vi "Volt Reader Trigger7.vi"() -> ()   [LabVIEW 2014]
uses:
  <vilib>/Utility/error.llb/DialogType.ctl
  <vilib>/_DAQmxBase/Internals/DAQmxBase Create Channel (AI-Voltage-Basic).vi
  <vilib>/_DAQmxBase/Internals/DAQmxBase Timing (Sample Clock).vi
  <vilib>/measure/mamon.llb/Trigger Detection for 1 Channel.vi
  <vilib>/_DAQmxBase/Internals/DAQmxBase Read (Analog 2D DBL NChan NSamp).vi
  <vilib>/measure/NI_MAPro.lvlib
panel:
  in  "Polarity":bool
  out "size of output array":i32
  out "Buffer Full?":bool
  out "trigger location":dbl format="%#_2g"
  out "Waveform Graph 2":waveform(dbl)(graph)
  in  "Continue Graphing":bool
  in  "Knob amplifier":dbl
  in  "Enable Center":bool
  in  "Center Button":bool
  in  "Knob":dbl(knob) scale=0.0..1.0
  out "Waveform Graph":waveform(dbl)(graph)
  in  "Buffer (Seconds)":dbl
  out "Threshold":dbl
  in  "units":i32(ring)=10348 items=["Volts"=10348, "From Custom Scale"=10065]
  in  "stop":bool
  in  "physical channels":tag
  in  "maximum value":dbl=5.0 format="%0.2f"
  in  "minimum value":dbl=-5.0 format="%0.2f"
  in  "rate":i32=1000 caption="Sample Rate"
  # "The inputs above MUST BE\nPreset before running"
  # "NOTE: Just change the Y axis value"
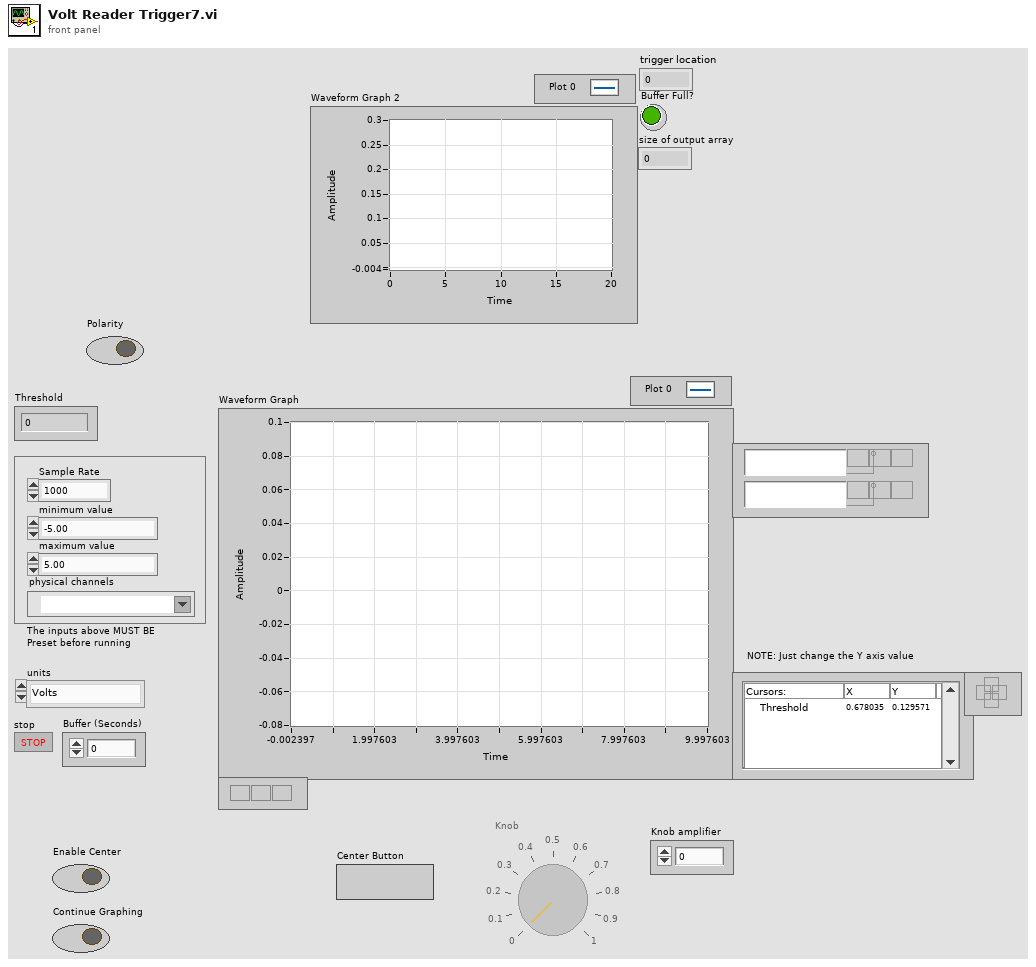
[diagram p1: front panel]
types:
  T1 = enum8{"Enabled", "Disabled", "Disabled and Grayed Out"}
  T2 = typedef "DialogType.ctl" = u16
  T3 = typedef "LVCursorListTypeDef.ctl" = cluster{"Name":string, "Color":u32, "Style":u8, "Point Style":u8, "Name Visible":bool, "Allow Drag":bool, "Cursor Mode":u32, "Plot":i32, "Index":i32, "Position":cluster{"X":dbl, "Y":dbl}, "X Scale":u32, "Y Scale":u32, "Watch Plots":i32[], "Watch All Plots":bool, "Plot Area":i32, "Label Offset":cluster{"X":dbl, "Y":dbl}}[]
  T4 = cluster{"Name":string, "Color":u32, "Style":u8, "Point Style":u8, "Name Visible":bool, "Allow Drag":bool, "Cursor Mode":u32, "Plot":i32, "Index":i32, "Position":cluster{"X":dbl, "Y":dbl}, "X Scale":u32, "Y Scale":u32, "Watch Plots":i32[], "Watch All Plots":bool, "Plot Area":i32, "Label Offset":cluster{"X":dbl, "Y":dbl}}
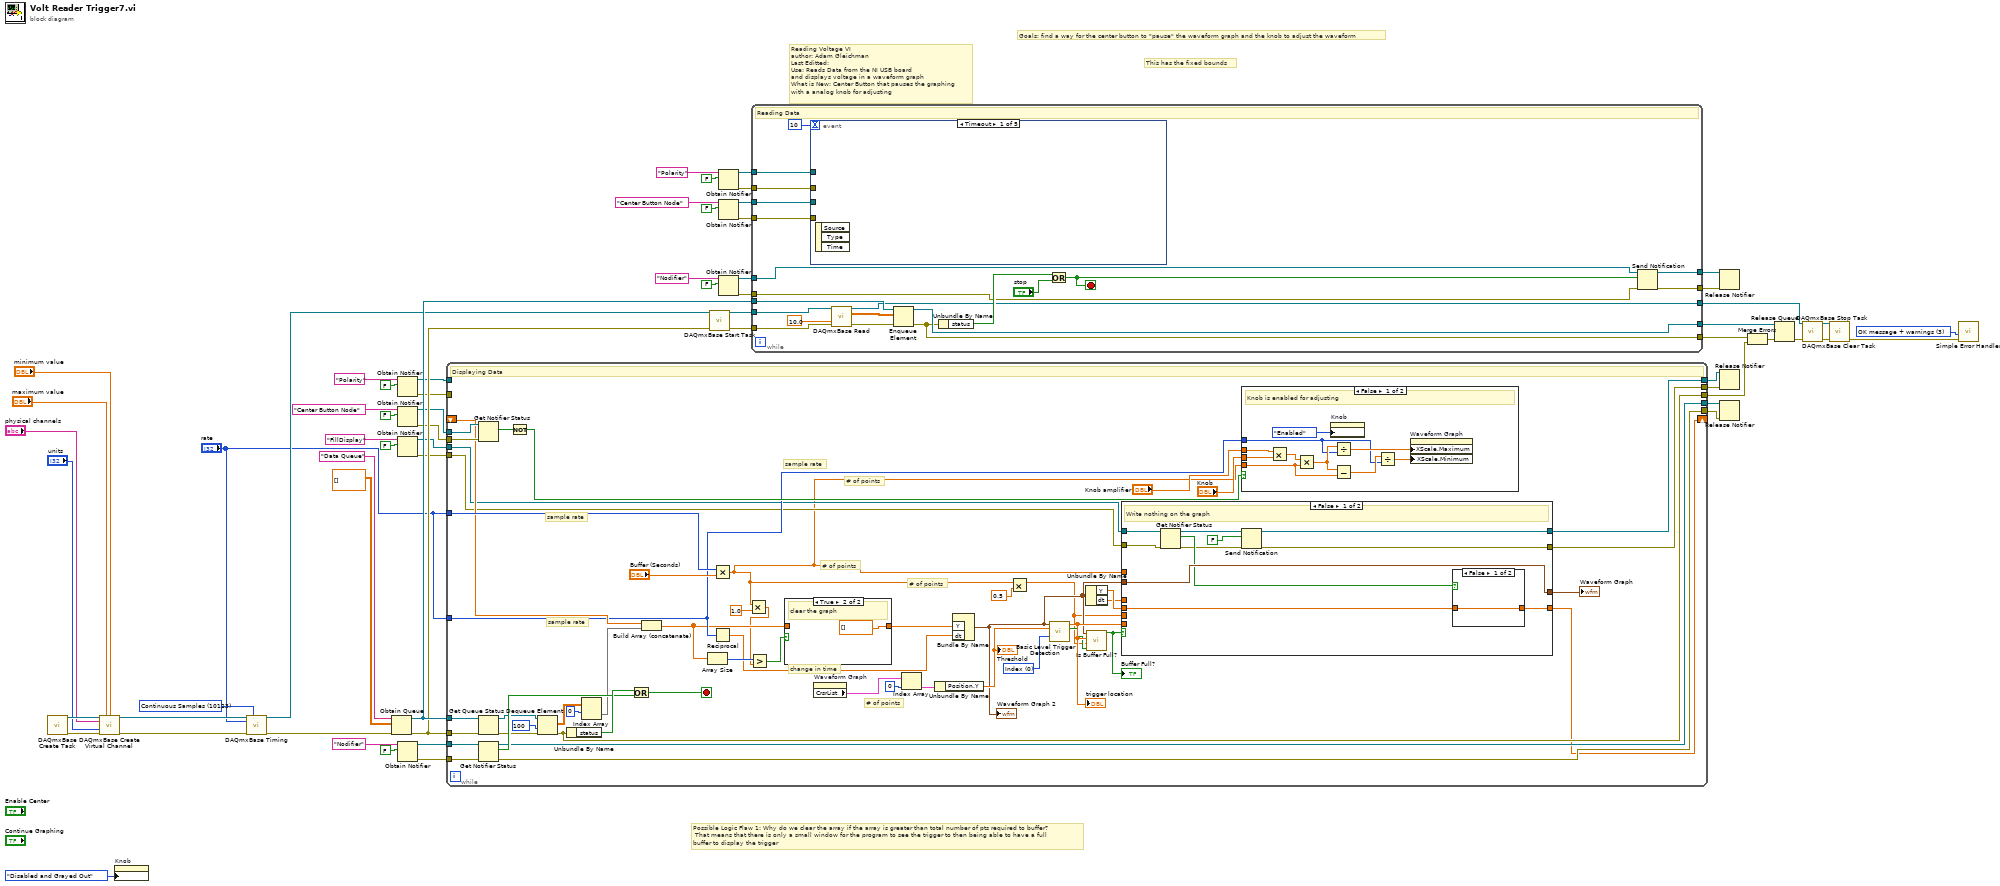
[diagram p0: block diagram]
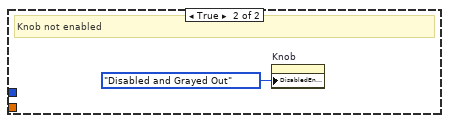
[diagram p3: hidden frame]
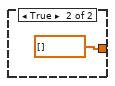
[diagram p4: hidden frame]
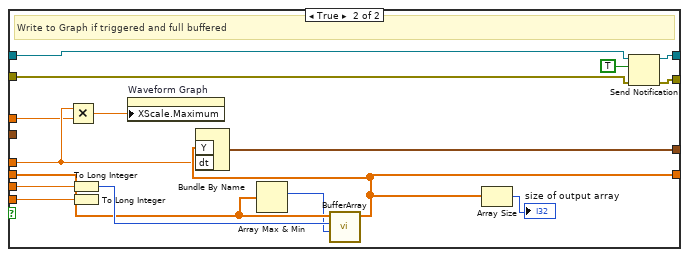
[diagram p5: hidden frame]
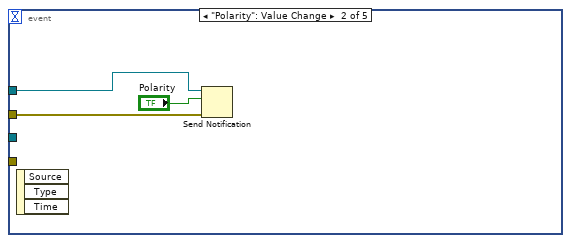
[diagram p6: hidden frame]
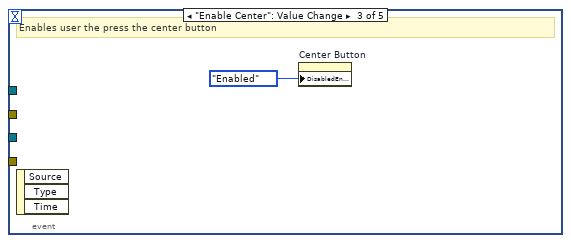
[diagram p7: hidden frame]
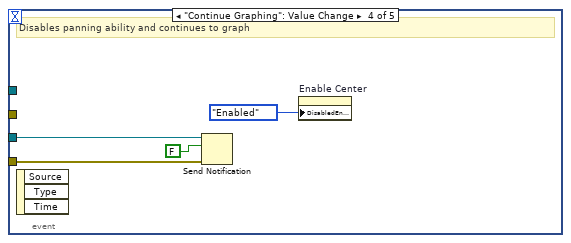
[diagram p8: hidden frame]
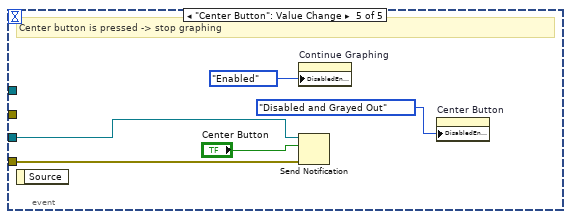
[diagram p9: hidden frame]
diagram:
  w40 = 10123 items=["Finite Samples"=10178, "Continuous Samples"=10123, "Hardware Timed Single Point"=12522] ("sample mode")
  w42 = T2 3 items=["no dialog", "OK message", "continue or stop message", "OK message + warnings", "continue/stop + warnings"] ("type of dialog (OK msg:1)")
  # "Possible Logic Flaw 1: Why do we clear the array if the array is greater than total number of pts required to buffer?\n That means that there is only a small window for the program to see the trigger to then being able to have a full\nbuffer to display the trigger"
  # "Goals: find a way for the center button to \"pause\" the waveform graph and the knob to adjust the waveform"
  # "This has the fixed bounds"
  # "Reading Voltage VI\nauthor: Adam Gleichman\nLast Editted: \nUse: Reads Data from the NI USB board\nand displays voltage in a waveform graph\nWhat is New: Center Button that pauses the graphing\nwith a analog knob for adjusting"
  n1 = call <vilib>:"DAQmxBase Create Task.vi"() -> ("task out"=w62:refnum<k21>, "error out"=w61:errorcluster)  [unwired: 5 in, 9 out]
  n2 = call-poly <vilib>:"DAQmxBase Create Virtual Channel.vi"("task in"=w62, "maximum value"="maximum value", "minimum value"="minimum value", "physical channels"="physical channels", "units"="units", "error in"=w61) -> ("task out"=w59:refnum<k21>, "error out"=w60:errorcluster)  [unwired: 3 in, 5 out]
  n3 = property on="Knob" class="Knob (strict)"("DisabledEnum"=T1."Disabled and Grayed Out" ("Disabled")) -> ()  [unwired: 2 in, 2 out]
  n4 = call-poly <vilib>:"DAQmxBase Timing.vi"("task/channels in"=w59, "sample mode"=w40, "rate"="rate", "error in"=w60) -> ("task out"=w28:refnum<k21>, "error out"=w27:errorcluster)  [unwired: 3 in, 7 out]
  n5 = Obtain Queue(name (unnamed)="Data Queue", element data type=dbl[][] [] ("data"), error in (no error)=w27) -> (queue out=w49:refnum<queue>, error out=w48:errorcluster)  [unwired: 2 in, 1 out]
  n6 = Obtain Notifier(name (unnamed)="Polarity", notification data type=FALSE) -> (notifier out=w8:refnum<notifier>, error out=w7:errorcluster)  [unwired: 2 in, 1 out]
  n7 = Obtain Notifier(name (unnamed)="Center Button Node", notification data type=FALSE) -> (notifier out=w15:refnum<notifier>, error out=w19:errorcluster)  [unwired: 2 in, 1 out]
  n8 = Obtain Notifier(name (unnamed)="FillDisplay", notification data type=FALSE) -> (notifier out=w6:refnum<notifier>, error out=w5:errorcluster)  [unwired: 2 in, 1 out]
  n9 = Obtain Notifier(name (unnamed)="Nodifier", notification data type=FALSE) -> (notifier out=w33:refnum<notifier>, error out=w31:errorcluster)  [unwired: 2 in, 1 out]
  n10 = while {
    tunnel: w49 -> [w116]
    tunnel: w48 -> [w105]
    tunnel: [w114] -> w47
    tunnel: w33 -> [w111]
    tunnel: w31 -> [w110]
    tunnel: [w108] -> w29
    tunnel: [w107] -> w30
    tunnel: "rate" -> [w81]
    tunnel: "rate" -> [w97]
    tunnel: w15 -> [w92]
    tunnel: w19 -> [w96]
    shift-right: [w89] -> _
    shift-left: _ -> [w88]
    tunnel: w8 -> [_]
    tunnel: w7 -> [_]
    tunnel: w6 -> [w78]
    tunnel: w5 -> [w77]
    tunnel: [w76] -> w2
    tunnel: [w75] -> w1
    stop <- w112 stop-if-true
    w86 = u16 0 items=["Index", "Time"] ("location mode")
    # "sample rate"
    # "# of points"
    # "change in time"
    # "# of points"
    # "# of points"
    # "# of points"
    # "sample rate"
    # "sample rate"
    # "Displaying Data"
    n11 = Get Notifier Status(notifier=w92, error in (no error)=w96) -> (current notification=w95:bool)  [unwired: 4 out]
    n12 = Get Queue Status(queue=w116, error in (no error)=w105) -> (queue out=w106:refnum<queue>, error out=w104:errorcluster)  [unwired: 1 in, 6 out]
    n13 = Get Notifier Status(notifier=w111, error in (no error)=w110) -> (notifier out=w108:refnum<notifier>, current notification=w109:bool, error out=w107:errorcluster)  [unwired: 2 out]
    n14 = Not(x=w95) -> (.not. x?=w93:bool)
    n15 = Dequeue Element(queue=w106, timeout in ms (-1)=100, error in (no error)=w104) -> (element=w102:dbl[][], error out=w114:errorcluster)  [unwired: 2 out]
    n16 = Unbundle By Name(w114) -> ("status"=w113:bool)
    n17 = Index Array(array=w102, index (row)=0 ("index")) -> (element=w90:dbl[])  [unwired: 1 in]
    n18 = Or(x=w113, y=w109) -> (x .or. y?=w112:bool)
    n19 = Build Array (concatenate)(w88, w90) -> (w71:dbl[])
    n20 = Array Size(array=w71) -> (size(s)=w74:i32)
    n21 = Multiply(x=w97, y="Buffer (Seconds)") -> (x*y=w68:dbl)
    n22 = Reciprocal(x=w81) -> (1/x=w70:dbl)
    n23 = Multiply(x=w68, y=1.0) -> (x*y=w66:dbl)
    n24 = Greater?(x=w74, y=w66) -> (0:w73:bool)
    n25 = case shown="True" w73 {
      tunnel: [w117 dbl[] []] -> w72
      tunnel: w71 -> [w117 _]
      frame False {
        # "does not exceed max points"
      }
      frame True {
        # "clear the graph"
      }
    }
    n26 = property on="Waveform Graph" class="WFGraph (strict)"() -> ("CrsrList"=w100:T3)  [unwired: 2 in, 2 out]
    n27 = Index Array(array=w100, index=0) -> (element=w99:T4)
    n28 = Unbundle By Name(w99) -> ("Position.Y"=w87:dbl)
    "Threshold" <- w87
    n29 = Bundle By Name("Y"=w72, "dt"=w70) -> (w79:waveform(dbl))  [unwired: 1 in]
    "Waveform Graph 2" <- w79
    n30 = Multiply(x=w68, y=0.5) -> (x*y=w65:dbl)
    n31 = call-poly <vilib>:"Basic Level Trigger Detection.vi"("signal in"=w79, "level"=w87, "location mode"=w86) -> ("trigger location"=w84:dbl, "trigger detected?"=w69:bool)  [unwired: 10 in, 1 out]
    "trigger location" <- w84
    n32 = Unbundle By Name(w79) -> ("Y"=w83:dbl[], "dt"=w82:dbl)
    n33 = call "Is Buffer Full?.vi"("Triggered?"=w69, "Buffer in Points"=w65, "Index location"=w84, "output waveform"=w79) -> ("Buffer Full?"=w85:bool)  [unwired: 7 in]
    "Buffer Full?" <- w85
    n34 = case shown="False" w85 {
      tunnel: w65 -> [_ w158]
      tunnel: [w138 w150] -> w89
      tunnel: w84 -> [_ w156]
      tunnel: w83 -> [w139 w144]
      tunnel: w82 -> [_ w146]
      tunnel: w68 -> [_ w145]
      tunnel: [w140 w154] -> w80
      tunnel: w79 -> [w140 _]
      tunnel: w78 -> [w136 w153]
      tunnel: w77 -> [w137 w152]
      tunnel: [w131 w149] -> w76
      tunnel: [w130 w148] -> w75
      frame False {
        # "Write nothing on the graph"
        n35 = Get Notifier Status(notifier=w136, error in (no error)=w137) -> (notifier out=w134:refnum<notifier>, current notification=w135:bool, error out=w133:errorcluster)  [unwired: 2 out]
        n36 = Send Notification(notification=FALSE, notifier=w134, error in (no error)=w133) -> (notifier out=w131:refnum<notifier>, error out=w130:errorcluster)
        n37 = case shown="False" w135 {
          tunnel: w139 -> [w141 _]
          tunnel: [w141 dbl[] []] -> w138
          frame False {
          }
          frame True {
          }
        }
      }
      frame True {
        # "Write to Graph if triggered and full buffered"
        n38 = Multiply(x=w146, y=w145) -> (x*y=w147:dbl)
        n39 = To Long Integer(number=w158) -> (32bit integer=w157:i32)
        n40 = To Long Integer(number=w156) -> ()  [unwired: 1 out]
        n41 = property on="Waveform Graph" class="WFGraph (strict)"("XScale.Maximum"=w147) -> ()  [unwired: 2 in, 2 out]
        n42 = Array Max & Min(array=w144) -> (max index (indices)=w143:i32)  [unwired: 3 out]
        n43 = call "BufferArray.vi"("Index"=w143, "Total amount of Pts"=w157, "Input Y-values"=w144) -> ("Output Array"=w150:dbl[])  [unwired: 8 in]
        n44 = Bundle By Name("Y"=w150, "dt"=w146) -> (w154:waveform(dbl))  [unwired: 1 in]
        n45 = Array Size(array=w150) -> (size(s)=→"size of output array":i32)
        n46 = Send Notification(notification=TRUE, notifier=w153, error in (no error)=w152) -> (notifier out=w149:refnum<notifier>, error out=w148:errorcluster)
      }
    }
    "Waveform Graph" <- w80
    n47 = case shown="False" w93 {
      tunnel: "Knob" -> [w126 _]
      tunnel: "Knob amplifier" -> [w127 _]
      tunnel: w68 -> [w124 _]
      tunnel: w81 -> [w119 _]
      frame False {
        # "Knob is enabled for adjusting"
        n48 = Multiply(x=w127, y=w126) -> (x*y=w125:dbl)
        n49 = Multiply(x=w125, y=w124) -> (x*y=w122:dbl)
        n50 = property on="Knob" class="Knob (strict)"("DisabledEnum"=T1."Enabled" ("Disabled")) -> ()  [unwired: 2 in, 2 out]
        n51 = Divide(x=w122, y=w119) -> (x/y=w120:dbl)
        n52 = Subtract(x=w122, y=w124) -> (x-y=w123:dbl)
        n53 = Divide(x=w123, y=w119) -> (x/y=w121:dbl)
        n54 = property on="Waveform Graph" class="WFGraph (strict)"("XScale.Maximum"=w120, "XScale.Minimum"=w121) -> ()  [unwired: 2 in, 2 out]
      }
      frame True {
        # "Knob not enabled"
        n55 = property on="Knob" class="Knob (strict)"("DisabledEnum"=T1."Disabled and Grayed Out" ("Disabled")) -> ()  [unwired: 2 in, 2 out]
      }
    }
  }
  n56 = call <vilib>:"DAQmxBase Start Task.vi"("task/channels in"=w28, "error in"=w48) -> ("task out"=w57:refnum<k21>, "error out"=w58:errorcluster)  [unwired: 12 out]
  n57 = Obtain Notifier(name (unnamed)="Polarity", notification data type=FALSE) -> (notifier out=w14:refnum<notifier>, error out=w13:errorcluster)  [unwired: 2 in, 1 out]
  n58 = Obtain Notifier(name (unnamed)="Center Button Node", notification data type=FALSE) -> (notifier out=w25:refnum<notifier>, error out=w24:errorcluster)  [unwired: 2 in, 1 out]
  n59 = Obtain Notifier(name (unnamed)="Nodifier", notification data type=FALSE) -> (notifier out=w36:refnum<notifier>, error out=w35:errorcluster)  [unwired: 2 in, 1 out]
  n60 = while "Data Reading Loop" {
    tunnel: w58 -> [w178]
    tunnel: w57 -> [w179]
    tunnel: w49 -> [w176]
    tunnel: [w173] -> w52
    tunnel: [w171] -> w51
    tunnel: [w169] -> w39
    tunnel: w36 -> [w167]
    tunnel: w35 -> [w166]
    tunnel: w25 -> [w165]
    tunnel: w24 -> [w164]
    tunnel: [w162] -> w17
    tunnel: [w161] -> w16
    tunnel: w14 -> [w160]
    tunnel: w13 -> [w159]
    stop <- w168 stop-if-true
    # "Reading Data"
    n61 = event shown="[0] Timeout" {
      selector: _ -> [_ _ _ _ _]
      dyn-events: _ -> [_ _ _ _ _]
      timeout: 10 -> [_ _ _ _ _]
      tunnel: w165 -> [_ _ _ w186 w192]
      tunnel: w164 -> [_ _ _ w185 w191]
      tunnel: w160 -> [_ w182 _ _ _]
      tunnel: w159 -> [_ w181 _ _ _]
      event Timeout {
        n62 = event-data() -> ()  [unwired: 1 in, 3 out]
      }
      event "Polarity": Value Change {
        n63 = event-data() -> ()  [unwired: 1 in, 3 out]
        n64 = Send Notification(notification="Polarity", notifier=w182, error in (no error)=w181) -> ()  [unwired: 2 out]
      }
      event "Enable Center": Value Change {
        # "Enables user the press the center button"
        n65 = event-data() -> ()  [unwired: 1 in, 3 out]
        n66 = property on="Center Button" class="Bool"("DisabledEnum"=T1."Enabled" ("Disabled")) -> ()  [unwired: 2 in, 2 out]
      }
      event "Continue Graphing": Value Change {
        # "Disables panning ability and continues to graph"
        n67 = event-data() -> ()  [unwired: 1 in, 3 out]
        n68 = Send Notification(notification=FALSE, notifier=w186, error in (no error)=w185) -> ()  [unwired: 2 out]
        n69 = property on="Enable Center" class="Bool (strict)"("DisabledEnum"=T1."Enabled" ("Disabled")) -> ()  [unwired: 2 in, 2 out]
      }
      event "Center Button": Value Change {
        # "Center button is pressed -> stop graphing"
        n70 = event-data() -> ()  [unwired: 1 in, 1 out]
        n71 = property on="Continue Graphing" class="Bool (strict)"("DisabledEnum"=T1."Enabled" ("Disabled")) -> ()  [unwired: 2 in, 2 out]
        n72 = Send Notification(notification="Center Button", notifier=w192, error in (no error)=w191) -> ()  [unwired: 2 out]
        n73 = property on="Center Button" class="Bool"("DisabledEnum"=T1."Disabled and Grayed Out" ("Disabled")) -> ()  [unwired: 2 in, 2 out]
      }
    }
    n74 = call-poly <vilib>:"DAQmxBase Read.vi"("task/channels in"=w179, "timeout"=10.0, "error in"=w178) -> ("task out"=w169:refnum<k21>, "data"=w174:dbl[][], "error out"=w177:errorcluster)  [unwired: 10 in]
    n75 = Enqueue Element(queue=w176, element=w174, error in (no error)=w177) -> (queue out=w173:refnum<queue>, error out=w171:errorcluster)  [unwired: 1 in, 1 out]
    n76 = Unbundle By Name(w171) -> ("status"=w170:bool)
    n77 = Or(x=w170, y="stop") -> (x .or. y?=w168:bool)
    n78 = Send Notification(notification=w168, notifier=w167, error in (no error)=w166) -> (notifier out=w162:refnum<notifier>, error out=w161:errorcluster)
  }
  n79 = Release Notifier(notifier=w17, error in (no error)=w16) -> ()  [unwired: 1 in, 3 out]
  n80 = Release Notifier(notifier=w2, error in (no error)=w1) -> ()  [unwired: 1 in, 3 out]
  n81 = Release Notifier(notifier=w29, error in (no error)=w30) -> ()  [unwired: 1 in, 3 out]
  n82 = Merge Errors(w51, w47) -> (w50:errorcluster)
  n83 = Release Queue(queue=w52, error in (no error)=w50) -> (error out=w46:errorcluster)  [unwired: 1 in, 2 out]
  n84 = call <vilib>:"DAQmxBase Stop Task.vi"("task/channels in"=w39, "error in"=w46) -> ("task out"=w45:refnum<k21>, "error out"=w44:errorcluster)  [unwired: 12 in]
  n85 = call <vilib>:"DAQmxBase Clear Task.vi"("task in"=w45, "error in"=w44) -> ("error out"=w43:errorcluster)  [unwired: 13 in]
  n86 = call <vilib>:"Simple Error Handler.vi"("type of dialog (OK msg:1)"=w42, "error in (no error)"=w43) -> ()  [unwired: 3 in, 5 out]
